vi "Config - Fire Command.vi"(8 "error in (no error)":errorcluster, 9 "Data":variant, 10 "CMD":T1, 11 "View Model":T2) -> (0 "error out":errorcluster, 3 "View Model":T2)   [LabVIEW 2017]
doc: "Generate user Event for send command to Config DB"
uses:
  View Model/Controls/View Model.ctl
  View Model/Controls/Shared Model.ctl
  Error Handler/Controls/Error Model.ctl
  Error Handler/Controls/Error Data.ctl
  Error Handler/Controls/Error Type.ctl
  Error Handler/Controls/Error Source.ctl
  Controls/Config Model.ctl
  Controls/Config CMD.ctl
  Controls/Config Command.ctl
  Controller/Controls/Controller Model.ctl
  Controller/Controls/Controller Overhead.ctl
  Controller/Controls/Controller Transaction.ctl
  Controller/Controls/Controller State.ctl
  Controls/Config Data Record.ctl
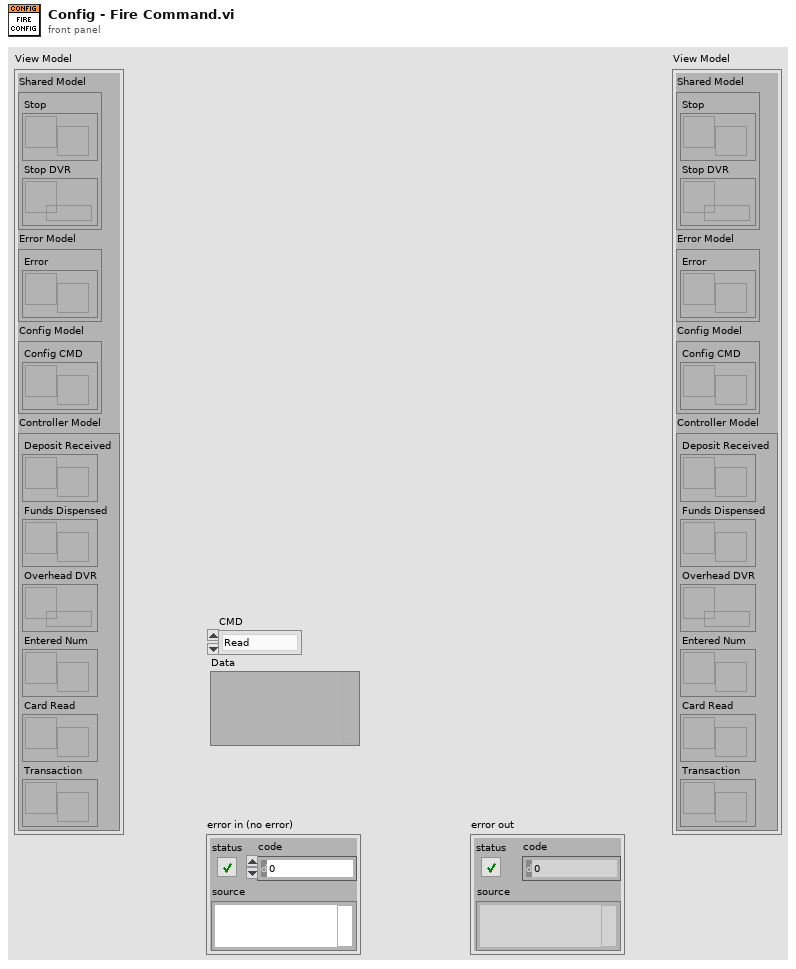
[diagram p1: front panel]
types:
  T1 = typedef "Config Command.ctl" = enum16{"Read", "Search", "Update"}
  T2 = typedef "View Model.ctl" = cluster{"Shared Model":T3, "Error Model":T4, "Config Model":T5, "Controller Model":T6}
  T3 = typedef "Shared Model.ctl" = cluster{"Stop":refnum<user-event>, "Stop DVR":refnum<data-value>}
  T4 = typedef "Error Model.ctl" = cluster{"Error":refnum<user-event>}
  T5 = typedef "Config Model.ctl" = cluster{"Config CMD":refnum<user-event>}
  T6 = typedef "Controller Model.ctl" = cluster{"Deposit Received":refnum<user-event>, "Funds Dispensed":refnum<user-event>, "Overhead DVR":refnum<data-value>, "Entered Num":refnum<user-event>, "Card Read":refnum<user-event>, "Transaction":refnum<user-event>}
  T7 = typedef "Config CMD.ctl" = cluster{"CMD":T1, "Data":variant}
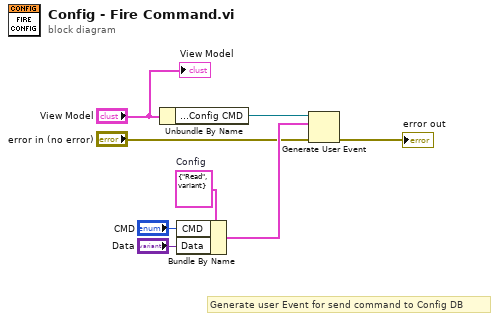
[diagram p0: block diagram]
diagram:
  w3 = T7 {"CMD"=enum."Read", "Data"=variant}  # Config
  # "Generate user Event for send command to Config DB"
  n1 = Unbundle By Name("View Model") -> ("Config Model.Config CMD"=w8:refnum<user-event>)
  n2 = Bundle By Name(cluster=w3, "CMD"="CMD", "Data"="Data") -> (w7:T7)
  n3 = Generate User Event(user event=w8, event data cluster=w7, error in="error in (no error)") -> (error out=→"error out":errorcluster)  [unwired: 1 in, 1 out]
  "View Model" <- "View Model"
